vi "Initialize.vi"(9 "Direction":T1, 10 "Job":T2(ring), 11 "Runner in":refnum<class "Cross.lvclass">) -> (3 "Runner out":refnum<class "Cross.lvclass">)   [LabVIEW 2015, in "Cross.lvclass"]
uses:
  Cross.lvclass
  Type Defs/Direction Enum.ctl
  Cross.lvclass/Cross.ctl
  Type Defs/SB Type Defs.lvlib
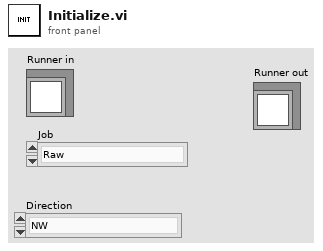
[diagram p1: front panel]
types:
  T1 = typedef "SB Type Defs.lvlib/Direction Enum.ctl" = enum16{"NW", "N", "NE", "E", "SE", "S", "SW", "W"}
  T2 = enum16{"Raw", "Spawner", "Builder", "Gunner", "Fighter"}
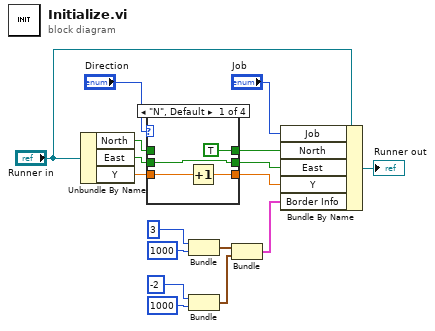
[diagram p0: block diagram]
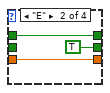
[diagram p2: hidden frame]
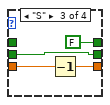
[diagram p3: hidden frame]
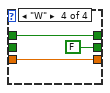
[diagram p4: hidden frame]
diagram:
  n1 = Unbundle By Name("Runner in") -> ("North"=w3:bool, "East"=w4:bool, "Y"=w6:dbl)
  n2 = case shown="\"N\", Default" "Direction" {
    tunnel: w6 -> [w21 w24 w28 w31]
    tunnel: [w20 w24 w27 w31] -> w5
    tunnel: w4 -> [w18 _ w26 _]
    tunnel: w3 -> [_ w23 _ w30]
    tunnel: [TRUE w23 FALSE w30] -> w2
    tunnel: [w18 TRUE w26 FALSE] -> w1
    frame "N", Default {
      n3 = Increment(x=w21) -> (x+1=w20:dbl)
    }
    frame "E" {
    }
    frame "S" {
      n4 = Decrement(x=w28) -> (x-1=w27:dbl)
    }
    frame "W" {
    }
  }
  n5 = Bundle(3, 1000) -> (w13:cluster{i32, i32})  [unwired: 1 in]
  n6 = Bundle(-2, 1000) -> (w12:cluster{i32, i32})  [unwired: 1 in]
  n7 = Bundle(w13, w12) -> (w10:cluster{cluster{i32, i32}, cluster{i32, i32}})  [unwired: 1 in]
  n8 = Bundle By Name(cluster="Runner in", "Job"="Job", "North"=w2, "East"=w1, "Y"=w5, "Border Info"=w10) -> (→"Runner out":refnum<class "Cross.lvclass">)
